vi "FPGA Main Default.vi"() -> ()   [LabVIEW 2016]
doc: "The myRIO v1.1 FPGA Shipping Personality. This personality contains support for:\n- 2 Analog Input Interrupt channel\n- 4 Digital Input Interrupt channel\n- 1 Timer\n- 1 Accelerometer\n- 1 Button\n- 4 LED\n- 10 Analog Input channels with 1 Sample\n- 6 Analog Output channels with 1 Sample\n- 40 Digital I/O channels with 1 Sample\n- 2 I2C channels\n- 4 Encoder channels\n- 6 PWM channels\n- 2 SPI channels"
uses:
  <vilib>/eio/EIONode/EIONode.xnode
  <vilib>/rvi/eio/common/nirviEmuTemplateMethod_errors.vi
panel:
  out "Numeric 2":i16
  out "Numeric":i16
  out "Waveform Chart 3":u16(graph)
  out "Waveform Chart 2":u16(graph)
  in  "AO.B_1.VAL":u16
  in  "AO.B_0.VAL":u16
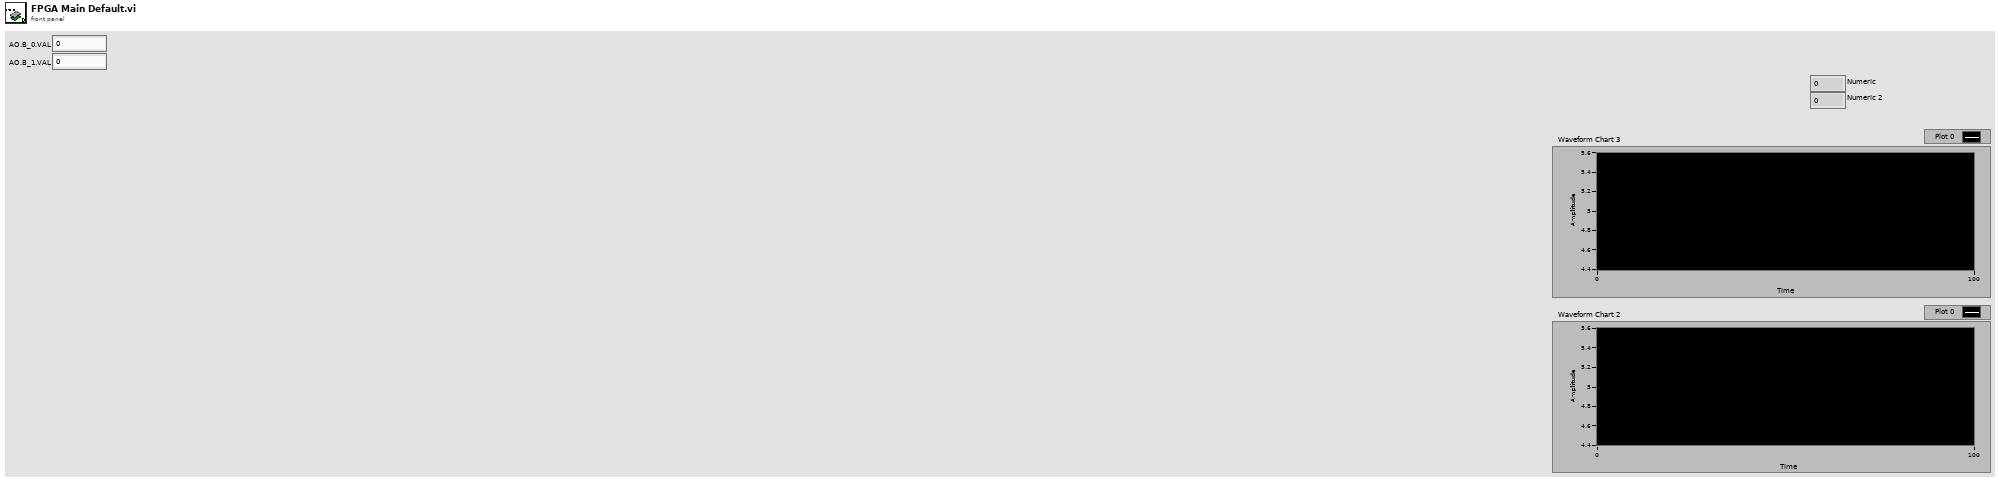
[diagram p1: front panel]
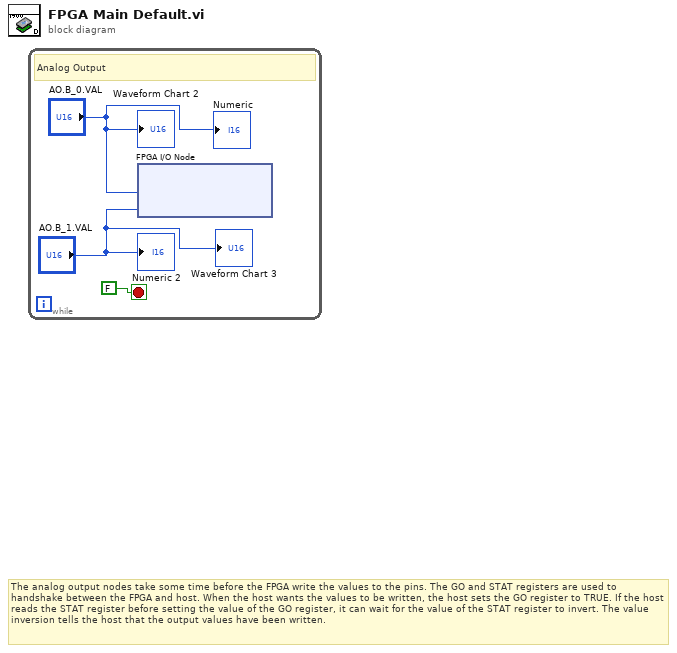
[diagram p0: block diagram]
diagram:
  # "The analog output nodes take some time before the FPGA write the values to the pins. The GO and STAT registers are used to handshake between the FPGA and host. When the host wants the values to be written, the host sets the GO register to TRUE. If the host reads the STAT register before setting the value of the GO register, it can wait for the value of the STAT register to invert. The value inversion tells the host that the output values have been written."
  n1 = while {
    stop <- FALSE stop-if-true
    # "Analog Output"
    n2 = xnode "FPGA I/O Node"("ConnectorB/AO0"="AO.B_0.VAL", "ConnectorB/AO1"="AO.B_1.VAL") -> ()  [unwired: 2 in, 2 out]
    "Waveform Chart 2" <- "AO.B_0.VAL"
    "Waveform Chart 3" <- "AO.B_1.VAL"
    "Numeric" <- "AO.B_0.VAL"
    "Numeric 2" <- "AO.B_1.VAL"
  }
